vi "Import Configuration RTM.vi"(8 "error in":errorcluster, 11 "Node Ptr":u64 format="%.0x") -> (0 "error out":errorcluster)   [LabVIEW 2020, in "Ballard ARINC 429 System Explorer.lvlib" / "Implementation.lvlib"]
uses:
  Implementation.lvlib
  Scripting/Ballard/Ballard ARINC 429 Scripting.lvlib
  Scripting/Ballard/Import Custom Device (In Place).vi
panel:
  in  "Tag":string
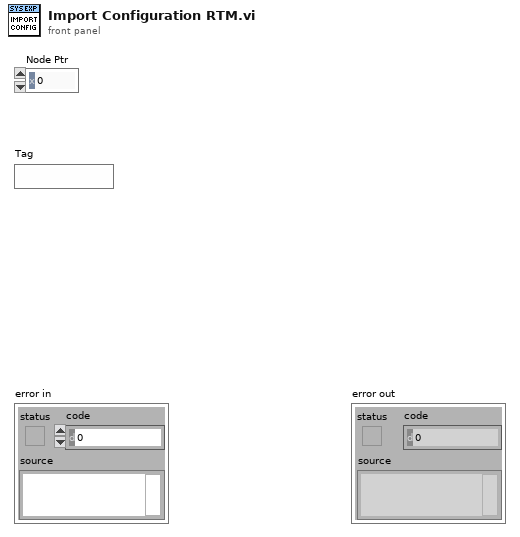
[diagram p1: front panel]
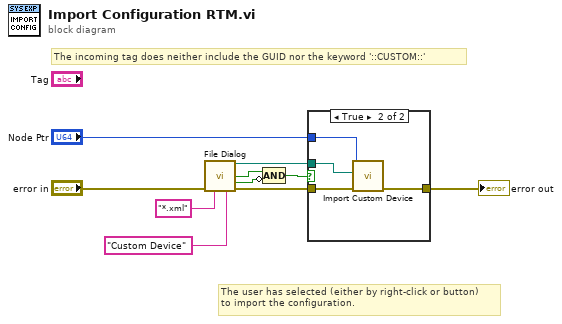
[diagram p0: block diagram]
diagram:
  # "The user has selected (either by right-click or button)\nto import the configuration."
  # "The incoming tag does neither include the GUID nor the keyword '::CUSTOM::'"
  n1 = call "File Dialog"("error in"="error in", "pattern (all files)"="*.xml" ("pattern label"), "pattern label"="Custom Device") -> ("selected path"=w4:path, "exists"=w9:bool, "cancelled"=w10:bool, "error out"=w5:errorcluster)  [unwired: 9 in]
  n2 = Compound Arithmetic op=AND(w9, invert w10) -> (w3:bool)
  n3 = case shown="True" w3 {
    tunnel: w5 -> [w11 w15]
    tunnel: w4 -> [_ w14]
    tunnel: "Node Ptr" -> [_ w13]
    tunnel: [w11 w12] -> w1
    frame False {
    }
    frame True {
      n4 = call-poly "Import Custom Device.vi"("error in"=w15, "path"=w14, "custom device ref"=w13) -> ("error out"=w12:errorcluster)  [unwired: 7 in, 1 out]
    }
  }
  "error out" <- w1
